vi "Read Potting Parameters.vi"(7 "Potting Surface Type":T1, 8 "error in":errorcluster, 11 "Config Manager in":refnum<class "Config Manager Class.lvclass">) -> (0 "error out":errorcluster, 2 "Potting Parameters":T2, 3 "Config Manager out":refnum<class "Config Manager Class.lvclass">)   [LabVIEW 2011, in "Config Manager Class.lvclass"]
uses:
  Config Manager Class.lvclass
  Type Definitions/Potting Parameters.ctl
  Type Definitions/Potting Surface Type.ctl
  Config Manager Class.lvclass/Config Manager Class.ctl
  <vilib>/Utility/config.llb/Read Key (Double).vi
  <vilib>/Utility/config.llb/NI_LVConfig.lvlib
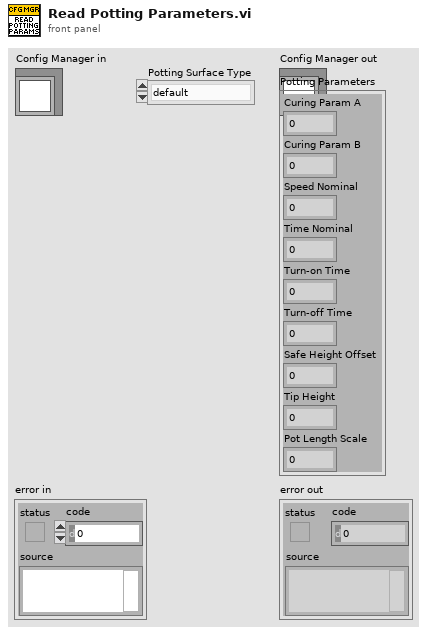
[diagram p1: front panel]
types:
  T1 = typedef "Potting Surface Type.ctl" = enum16{"default", "hdi_edge_pads"}
  T2 = typedef "Potting Parameters.ctl" = cluster{"Curing Param A":dbl, "Curing Param B":dbl, "Speed Nominal":dbl, "Time Nominal":dbl, "Turn-on Time":dbl, "Turn-off Time":dbl, "Safe Height Offset":dbl, "Tip Height":dbl, "Pot Length Scale":dbl}
  T3 = typedef "NI_LVConfig.lvlib/Config Data RefNum.ctl" = refnum<k1>
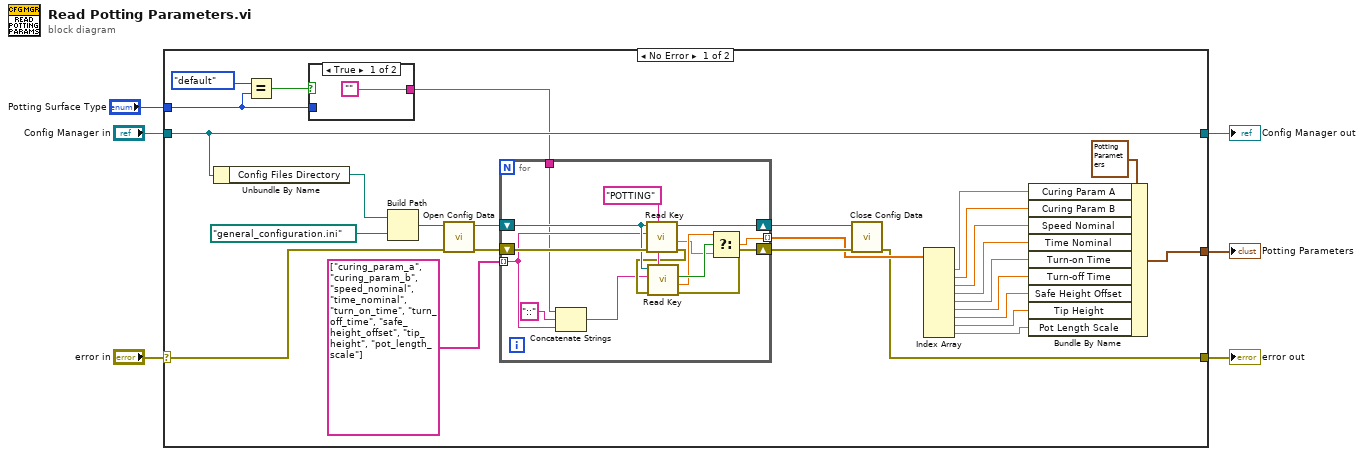
[diagram p0: block diagram]
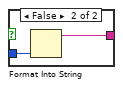
[diagram p2: hidden frame]
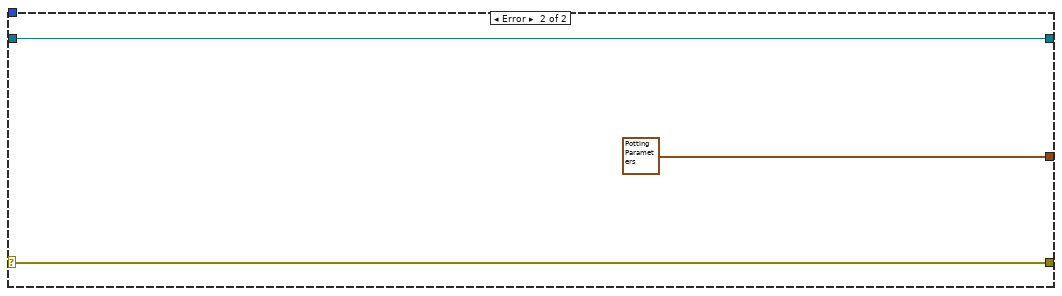
[diagram p3: hidden frame]
diagram:
  n1 = case shown="No Error" "error in" {
    selector: "error in" -> [w31 w53]
    tunnel: [w13 w53] -> w5
    tunnel: [w30 w52] -> w3
    tunnel: "Config Manager in" -> [w30 w52]
    tunnel: [w27 T2 {"Curing Param A"=0.0, "Curing Param B"=0.0, "Speed Nominal"=0.0, "Time Nominal"=0.0, "Turn-on Time"=0.0, "Turn-off Time"=0.0, "Safe Height Offset"=0.0, "Tip Height"=0.0, "Pot Length Scale"=0.0} ("Potting Parameters 2")] -> w2
    tunnel: "Potting Surface Type" -> [w10 _]
    frame No Error {
      n2 = Unbundle By Name(w30) -> ("Config Files Directory"=w29:path)
      n3 = Equal?(x=Potting_Surface_Type."default", y=w10) -> (x = y?=w11:bool)
      n4 = case shown="True" w11 {
        tunnel: ["" w35] -> w9
        tunnel: w10 -> [_ w36]
        frame True {
        }
        frame False {
          n5 = Format Into String(w36) -> (resulting string=w35:string)  [unwired: 3 in, 1 out]
        }
      }
      n6 = Build Path(base path=w29, name or relative path=path "general_configuration.ini") -> (appended path=w32:path)
      n7 = call <vilib>:"Open Config Data.vi"("error in (no error)"=w31, "configuration file path"=w32) -> ("error out"=w24:errorcluster, "refnum"=w25:T3)  [unwired: 7 in, 1 out]
      n8 = for {
        tunnel: string[] ["curing_param_a", "curing_param_b", "speed_nominal", "time_nominal", "turn_on_time", "turn_off_time", "safe_height_offset", "tip_height", "pot_length_scale"] -> [w46] mode=indexing
        shift-right: [w38] -> w22
        shift-left: w25 -> [w48]
        tunnel: [w39] -> w21 mode=indexing
        shift-right: [w37] -> w23
        shift-left: w24 -> [w50]
        tunnel: w9 -> [w45]
        w49 = "POTTING" ("section")
        n9 = Concatenate Strings(w45, "::" ("string"), w46) -> (w43:string)
        n10 = call-poly <vilib>:"Read Key.vi"("section"=w49, "error in (no error)"=w50, "key"=w46, "refnum"=w48) -> ("error out"=w47:errorcluster, "value"=w40:dbl, "refnum out"=w38:T3)  [unwired: 4 in, 1 out]
        n11 = call-poly <vilib>:"Read Key.vi"("section"=w49, "error in (no error)"=w47, "key"=w43, "refnum"=w48) -> ("error out"=w37:errorcluster, "value"=w41:dbl, "found?"=w42:bool)  [unwired: 4 in, 1 out]
        n12 = Select(t=w41, s=w42, f=w40) -> (s? t:f=w39:dbl)
      }
      n13 = call <vilib>:"Close Config Data.vi"("error in (no error)"=w23, "refnum"=w22) -> ("error out"=w13:errorcluster)  [unwired: 8 in, 1 out]
      n14 = Index Array(array=w21) -> (element #1=w20:dbl, element #2=w19:dbl, element #3=w18:dbl, element #4=w17:dbl, element #5=w16:dbl, element #6=w15:dbl, element #7=w14:dbl, element #8=w8:dbl, element #9=w7:dbl)  [unwired: 9 in]
      n15 = Bundle By Name(cluster=T2 {"Curing Param A"=0.0, "Curing Param B"=0.0, "Speed Nominal"=0.0, "Time Nominal"=0.0, "Turn-on Time"=0.0, "Turn-off Time"=0.0, "Safe Height Offset"=0.0, "Tip Height"=0.0, "Pot Length Scale"=0.0} ("Potting Parameters 2"), "Curing Param A"=w20, "Curing Param B"=w19, "Speed Nominal"=w18, "Time Nominal"=w17, "Turn-on Time"=w16, "Turn-off Time"=w15, "Safe Height Offset"=w14, "Tip Height"=w8, "Pot Length Scale"=w7) -> (w27:T2)
    }
    frame Error {
    }
  }
  "error out" <- w5
  "Config Manager out" <- w3
  "Potting Parameters" <- w2
